vi "Encoder RPM.vi"(11 "Encoder Rate":dbl) -> (3 "Encoder RPM":dbl)   [LabVIEW 2011]
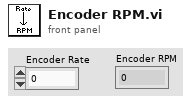
[diagram p1: front panel]
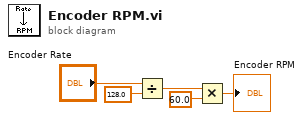
[diagram p0: block diagram]
diagram:
  n1 = Divide(x="Encoder Rate", y=128.0) -> (x/y=w3:dbl)
  n2 = Multiply(x=w3, y=60.0) -> (x*y=→"Encoder RPM":dbl)
